vi "Do.vi"(8 "error in (no error)":errorcluster, 10 "Actor in":refnum<class "Actor.lvclass">, 11 "Measurement Done":refnum<class "Measurement Done.lvclass">) -> (0 "error out":errorcluster, 2 "Actor out":refnum<class "Actor.lvclass">)   [LabVIEW 2017, in "Controller Actor.lvlib" / "Measurement Done.lvclass"]
uses:
  Measurement Done.lvclass
  <vilib>/ActorFramework/Actor/Actor.lvclass
  Controller.lvclass
  C:/Program Files (x86)/National Instruments/LabVIEW 2017/vi.lib/ActorFramework/Actor/Actor.lvclass
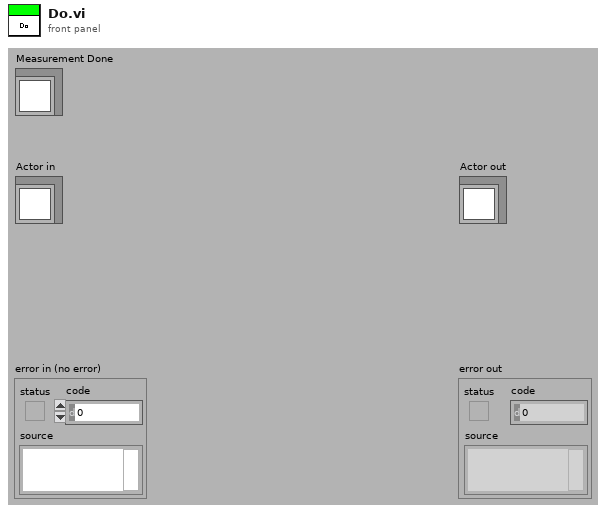
[diagram p1: front panel]
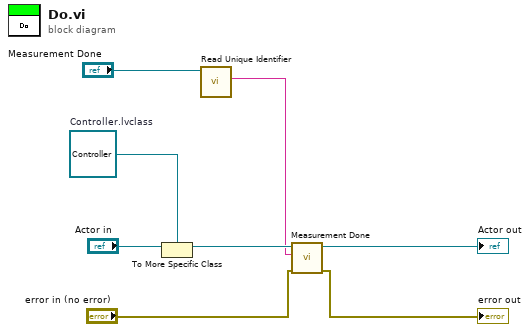
[diagram p0: block diagram]
diagram:
  w3 = refnum<class "Controller.lvclass"> refnum  # Controller.lvclass
  n1 = To More Specific Class(target class=w3, reference="Actor in") -> (specific class reference=w7:refnum<class "Controller.lvclass">)  [unwired: 1 in, 1 out]
  n2 = call "Read Unique Identifier.vi"("Measurement Done in"="Measurement Done") -> ("Unique Identifier"=w5:string)  [unwired: 8 in, 2 out]
  n3 = call-dynamic "Measurement Done.vi"("error in (no error)"="error in (no error)", "GUID"=w5, "Controller in"=w7) -> ("error out"=→"error out":errorcluster, "Controller out"=→"Actor out":refnum<class "Controller.lvclass">)  [unwired: 7 in]
